vi "MTM2_getEvent_settingsApplied.vi"(8 "error in (no error)":errorcluster, 11 "logevent_settingsApplied_Ctl":T1={"private_rcvStamp"=0.0, "settingsVersion"="                                                                                                                                                                                                                                                                ", "otherSettingsEvents"="", "priority"=0}) -> (0 "error out":errorcluster, 2 "function return":i32, 3 "logevent_settingsApplied_Ctl out":T1={"private_rcvStamp"=0.0, "settingsVersion"="                                                                                                                                                                                                                                                                ", "otherSettingsEvents"="", "priority"=0})   [LabVIEW 2018, in "SALLV_MTM2.lvlib"]
doc: "int MTM2_shm_getEvent_settingsAppliedLV(MTM2_logevent_settingsAppliedLV *logevent_settingsApplied_Ctl );"
uses:
  DataTypes/logevent_settingsApplied.ctl
  SALLV_MTM2.lvlib
  SALLV_MTM2.so
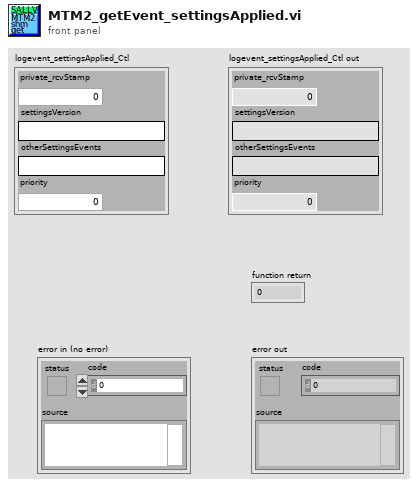
[diagram p1: front panel]
types:
  T1 = typedef "SALLV_MTM2.lvlib/logevent_settingsApplied.ctl" = cluster{"private_rcvStamp":dbl, "settingsVersion":string, "otherSettingsEvents":string, "priority":i32}
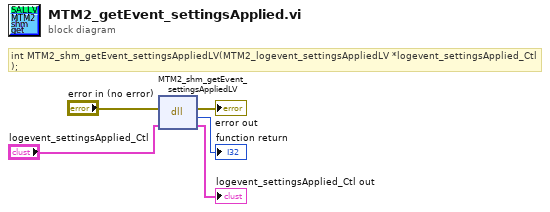
[diagram p0: block diagram]
diagram:
  # "int MTM2_shm_getEvent_settingsAppliedLV(MTM2_logevent_settingsAppliedLV *logevent_settingsApplied_Ctl );"
  n1 = dll-call lib="home/ttsai/Documents/salLabviewApi/SALLV_MTM2/SALLV_MTM2.*" fn="MTM2_shm_getEvent_settingsAppliedLV"(error in="error in (no error)", "logevent_settingsApplied_Ctl"="logevent_settingsApplied_Ctl") -> (error out=→"error out":errorcluster, →"function return":i32, "logevent_settingsApplied_Ctl"=→"logevent_settingsApplied_Ctl out":T1)  [unwired: 2 in, 1 out]
